vi "Acquire Class Details_Variant.vi"(8 "error in":errorcluster, 11 "Class Path":path) -> (0 "error out":errorcluster, 1 "Member VI info":T1[](array[typedef]), 2 "Interface file names":string[](array[string]), 3 "Hierarchy":string[](array[string]))   [LabVIEW 2019]
uses:
  <vilib>/Utility/Data Type/NI_Data Type.lvlib
  <vilib>/Utility/Data Type/Member VI Info.ctl
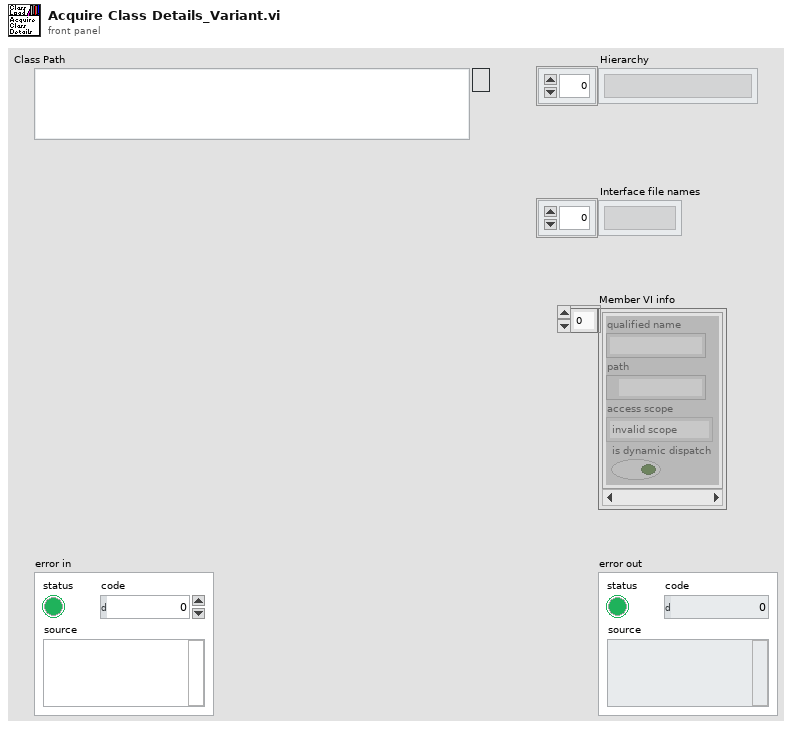
[diagram p1: front panel]
types:
  T1 = typedef "Member VI Info.ctl" = cluster{"qualified name":string, "path":path, "access scope":enum32{"invalid scope", "public", "private", "protected", "community"}, "is dynamic dispatch":bool}
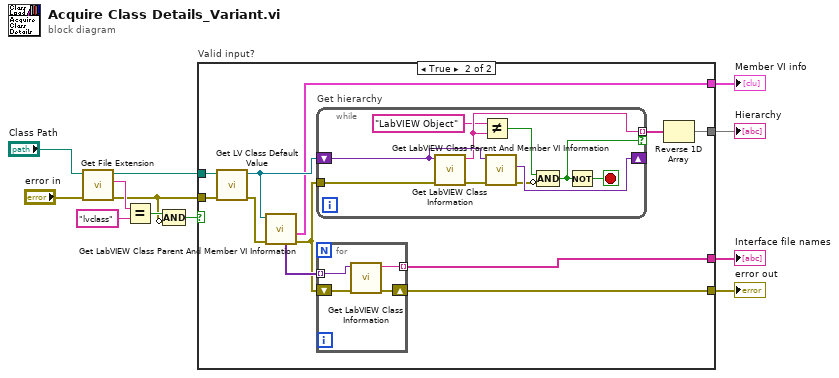
[diagram p0: block diagram]
diagram:
  n1 = call <vilib>:"Get File Extension.vi"("error in (no error)"="error in", "file"="Class Path") -> ("error out"=w5:errorcluster, "lowercase file extension"=w11:string, "dup file"=w4:path)  [unwired: 5 in, 2 out]
  n2 = Equal?(x=w11, y="lvclass" ("x")) -> (x = y?=w9:bool)
  n3 = Compound Arithmetic op=AND(w9, invert w5) -> (w7:bool)
  n4 = case "Valid input?" shown="True" w7 {
    tunnel: [w13 w15] -> w6
    tunnel: w5 -> [w13 w23]
    tunnel: w4 -> [_ w24]
    tunnel: [_ w21] -> w3
    tunnel: [_ w18] -> w2
    tunnel: [_ w14] -> w1
    frame False {
    }
    frame True {
      n5 = call <vilib>:"Get LV Class Default Value.vi"("error in (no error)"=w23, "class path"=w24) -> ("error out"=w19:errorcluster, "object"=w20:refnum<class>)  [unwired: 8 in]
      n6 = call <vilib>:"Get LabVIEW Class Parent And Member VI Information.vi"("error in (no error)"=w19, "variant"=w20) -> ("error out"=w16:errorcluster, "member VI info"=w18:T1[], "parent interfaces"=w17:variant[])  [unwired: 6 in, 1 out]
      n7 = while "Get hierarchy" {
        shift-right: [w38] -> _
        shift-left: w20 -> [w37]
        tunnel: w16 -> [w35]
        tunnel: [w34] -> w22 mode=indexing if=w30
        stop <- w29 stop-if-true
        n8 = call <vilib>:"Get LabVIEW Class Information.vi"("error in (no error)"=w35, "variant"=w37) -> ("error out"=w36:errorcluster, "LabVIEW class file name"=w34:string)  [unwired: 7 in, 1 out]
        n9 = Not Equal?(x="LabVIEW Object" ("y"), y=w34) -> (x != y?=w32:bool)
        n10 = call <vilib>:"Get LabVIEW Class Parent And Member VI Information.vi"("error in (no error)"=w36, "variant"=w37) -> ("error out"=w31:errorcluster, "parent class"=w38:variant)  [unwired: 6 in, 2 out]
        n11 = Compound Arithmetic op=AND(w32, invert w31) -> (w30:bool)
        n12 = Not(x=w30) -> (.not. x?=w29:bool)
      }
      n13 = for {
        tunnel: w17 -> [w28] mode=indexing
        shift-right: [w26] -> w15
        shift-left: w16 -> [w27]
        tunnel: [w25] -> w14 mode=indexing
        n14 = call <vilib>:"Get LabVIEW Class Information.vi"("error in (no error)"=w27, "variant"=w28) -> ("error out"=w26:errorcluster, "LabVIEW class file name"=w25:string)  [unwired: 7 in, 1 out]
      }
      n15 = Reverse 1D Array(array=w22) -> (reversed array=w21:string[])
    }
  }
  "error out" <- w6
  "Hierarchy" <- w3
  "Member VI info" <- w2
  "Interface file names" <- w1
